vi "Configure DIO Direction.vi"(0 "RedPitaya connection in":refnum<k5>, 2 "Pin #":string, 3 "Direction":string(combo), 5 "error in":errorcluster, 12 "timeout ms (2000)":i32=2000) -> (14 "RedPitaya connection out":refnum<k5>, 19 "error out":errorcluster)   [LabVIEW 2010, in "RedPitaya.lvlib"]
doc: "Set direction of digital pins to output or input."
uses:
  RedPitaya.lvlib
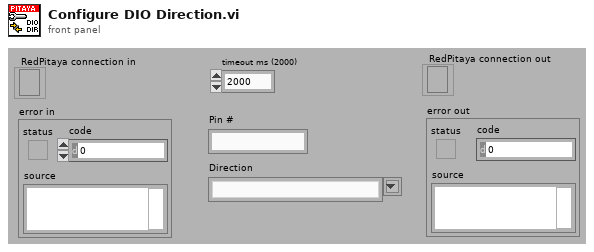
[diagram p1: front panel]
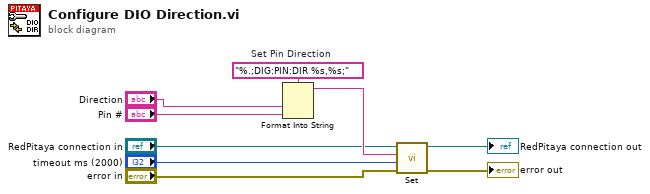
[diagram p0: block diagram]
diagram:
  w9 = "%.;DIG:PIN:DIR %s,%s;"  # Set Pin Direction
  n1 = Format Into String(format string=w9, "Direction", "Pin #") -> (resulting string=w8:string)  [unwired: 2 in, 1 out]
  n2 = call "Set.vi"("error in"="error in", "timeout ms (2000)"="timeout ms (2000)", "SCPI Message"=w8, "RedPitaya connection in"="RedPitaya connection in") -> ("error out"=→"error out":errorcluster, "RedPitaya connection out"=→"RedPitaya connection out":refnum<k5>)  [unwired: 5 in, 1 out]
